vi "FP_CtrlEnable (SubVI).vi"(8 "error in":errorcluster, 10 "Disabled":T1(ring), 11 "Array":refnum<vi>[](array[refnum])) -> (0 "error out":errorcluster)   [LabVIEW 2017]
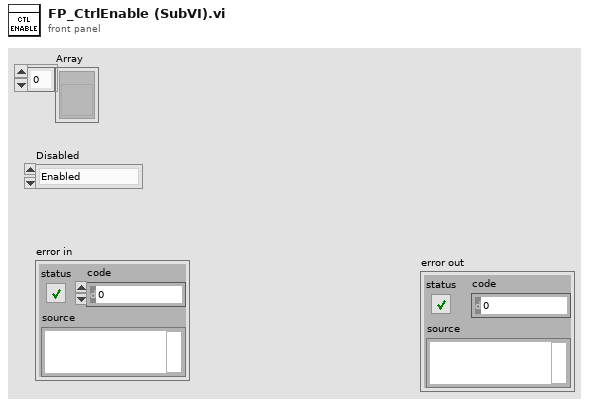
[diagram p1: front panel]
types:
  T1 = enum8{"Enabled", "Disabled", "Disabled and Grayed Out"}
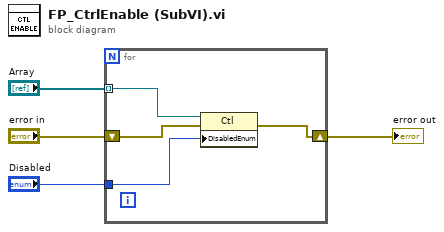
[diagram p0: block diagram]
diagram:
  n1 = for {
    tunnel: "Disabled" -> [w8]
    tunnel: "Array" -> [w7] mode=indexing
    shift-right: [w5] -> w1
    shift-left: "error in" -> [w6]
    n2 = property on="Property Node" class="Ctl"(reference=w7, error in=w6, "DisabledEnum"=w8) -> (error out=w5:errorcluster)  [unwired: 1 out]
  }
  "error out" <- w1
